vi "VisOpticsErrCodesDetector.vi"(2 "error in":errorcluster) -> (3 "NHMFL Visible Optics Error Category":T2, 4 "Error Category text":string, 5 "NHMFL Visible Optics Error Type":T1(ring), 6 "Error Type text":string)   [LabVIEW 2019]
doc: "This is to generate user-defined error codes, to be used as Typre-Defs:\nNHMFL Visible Optics Error Categories\nNHMFL Visible Optics Error Type\nNHMFL Visible Optics user-defined error codes\nNHMFL Visible Optics user-defined error descriptions"
uses:
  Globals and TypeDefs/Error Categories.ctt
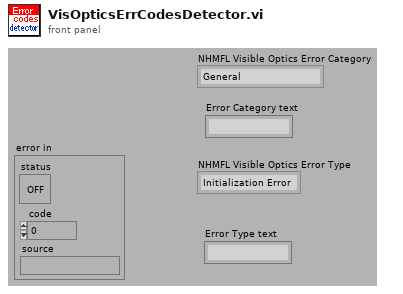
[diagram p1: front panel]
types:
  T1 = enum8{"Initialization Error", "Command Error", "Parameter Error", "Overflow Error", "Time-out Error", "Misc Error", "User cancel"}
  T2 = typedef "Error Categories.ctt" = enum8{"General", "CCD-256x1024", "CCD-1340x400", "InGaAs PDA", "McPherson 2075", "Magnetic Field", "Temperature Control", "Other"}
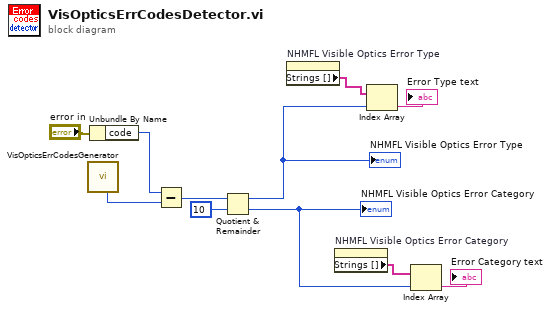
[diagram p0: block diagram]
diagram:
  n1 = call "VisOpticsErrCodesGenerator.vi"() -> ("Error Code base number output"=w11:i32)  [unwired: 3 in, 5 out]
  n2 = Unbundle By Name("error in") -> ("code"=w1:i32)
  n3 = Subtract(x=w1, y=w11) -> (x-y=w10:i32)
  n4 = Quotient & Remainder(x=w10, y=10) -> (x-y*floor(x/y)=w3:i32, floor(x/y)=w7:i32)
  "NHMFL Visible Optics Error Category" <- w7
  "NHMFL Visible Optics Error Type" <- w3
  n5 = property on="NHMFL Visible Optics Error Type" class="Enum (strict)"() -> ("Strings []"=w4:string[])  [unwired: 2 in, 2 out]
  n6 = property on="NHMFL Visible Optics Error Category" class="Enum (strict)"() -> ("Strings []"=w8:string[])  [unwired: 2 in, 2 out]
  n7 = Index Array(array=w4, index=w3) -> (element=→"Error Type text":string)
  n8 = Index Array(array=w8, index=w7) -> (element=→"Error Category text":string)
